vi "recentMax.vi"(8 "MemLen":i32, 11 "Input":dbl) -> (3 "Input 2":dbl)   [LabVIEW 2010, in "KevLib01.lvlib"]
uses:
  KevLib01.lvlib
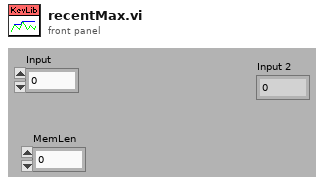
[diagram p1: front panel]
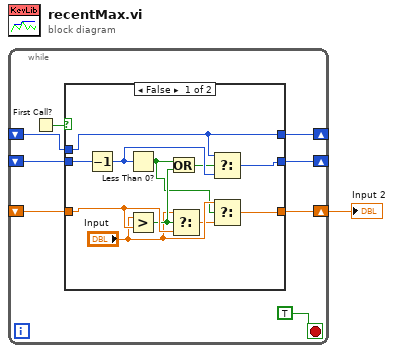
[diagram p0: block diagram]
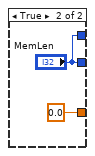
[diagram p2: hidden frame]
diagram:
  n1 = while {
    shift-right: [w7] -> _
    shift-left: _ -> [w6]
    shift-right: [w4] -> _
    shift-left: _ -> [w5]
    shift-right: [w3] -> w1
    shift-left: _ -> [w2]
    stop <- TRUE stop-if-true
    n2 = First Call?() -> (First Call?: T/F=w8:bool)
    n3 = case shown="False" w8 {
      tunnel: [w19 "MemLen"] -> w7
      tunnel: w6 -> [w19 _]
      tunnel: w5 -> [w20 _]
      tunnel: [w18 "MemLen"] -> w4
      tunnel: [w11 0.0 ("Input")] -> w3
      tunnel: w2 -> [w16 _]
      frame False {
        n4 = Decrement(x=w20) -> (x-1=w17:i32)
        n5 = Less Than 0?(x=w17) -> (x < 0?=w10:bool)
        n6 = Greater?(x="Input", y=w16) -> (0:w15:bool)
        n7 = Or(x=w10, y=w15) -> (x .or. y?=w14:bool)
        n8 = Select(t="Input", s=w15, f=w16) -> (s? t:f=w12:dbl)
        n9 = Select(t=w19, s=w14, f=w17) -> (s? t:f=w18:i32)
        n10 = Select(t="Input", s=w10, f=w12) -> (s? t:f=w11:dbl)
      }
      frame True {
      }
    }
  }
  "Input 2" <- w1
